vi "MatrixSwitchSingle.vi"(7 "Switch action":u16(ring) items=["Open", "Close"], 8 "error in (no error)":errorcluster, 9 "Matrix Y":i32=1 min=1 max=12 step=1, 10 "Matrix X":i32=1 min=1 max=12 step=1, 11 "LXIPXISwitching in":refnum<class "LXIPXISwitching.lvclass">) -> (0 "error out":errorcluster, 2 "command string":string, 3 "LXIPXISwitching out":refnum<class "LXIPXISwitching.lvclass">)   [LabVIEW 2019, in "LXIPXISwitching.lvclass"]
uses:
  LXIPXISwitching.lvclass
  InstrumentSetup.vi
  InstrControl.lvclass
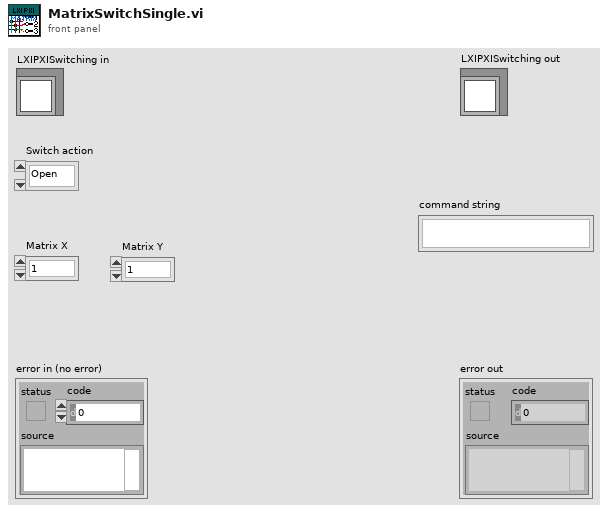
[diagram p1: front panel]
types:
  T1 = cluster{"MUX":string, "Matrix":string, "Breadboard":string, "LXIPXI Switching":refnum<class "LXIPXISwitching.lvclass">, "MUX PN":string, "Matrix  PN":string, "Breadboard PN":string, "MUX ID":string, "Matrix ID":string, "Breadboard ID":string, "LCR?":bool, "SMU?":bool}
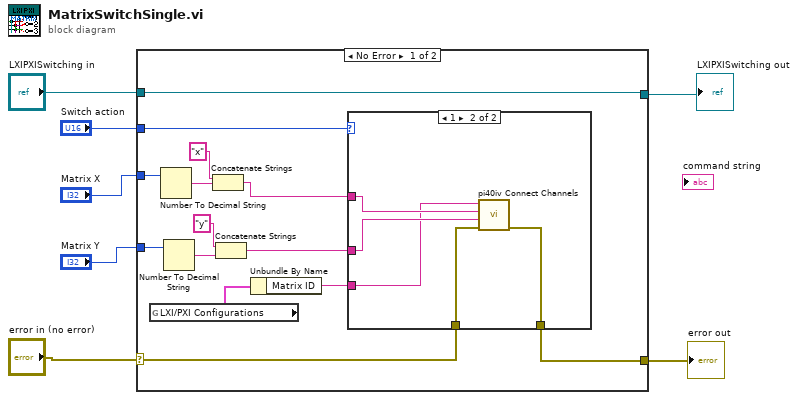
[diagram p0: block diagram]
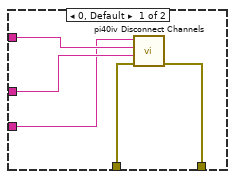
[diagram p2: hidden frame]
diagram:
  n1 = case shown="No Error" "error in (no error)" {
    selector: "error in (no error)" -> [w11 w33]
    tunnel: [w10 w33] -> w6
    tunnel: [w21 w32] -> w4
    tunnel: "LXIPXISwitching in" -> [w21 w32]
    tunnel: "Switch action" -> [w20 _]
    tunnel: "Matrix X" -> [w19 _]
    tunnel: "Matrix Y" -> [w18 _]
    frame No Error {
      n2 = global read "InstrumentSetup.vi" "LXI/PXI Configurations"() -> (w9:T1)
      n3 = Number To Decimal String(number=w19) -> (decimal integer string=w15:string)  [unwired: 1 in]
      n4 = Number To Decimal String(number=w18) -> (decimal integer string=w14:string)  [unwired: 1 in]
      n5 = Concatenate Strings("x" ("string"), w15) -> (w12:string)
      n6 = Concatenate Strings("y" ("string"), w14) -> (w13:string)
      n7 = Unbundle By Name(w9) -> ("Matrix ID"=w8:string)
      n8 = case shown="1" w20 {
        tunnel: w13 -> [w26 w30]
        tunnel: w12 -> [w25 w31]
        tunnel: w11 -> [w24 w29]
        tunnel: [w23 w28] -> w10
        tunnel: w8 -> [w22 w27]
        frame 0, Default {
          n9 = call <instrlib>:"pi40iv Disconnect Channels.vi"("error in (no error)"=w24, "channel 2"=w26, "channel 1"=w25, "instrument handle"=w22) -> ("error out"=w23:errorcluster)  [unwired: 6 in, 1 out]
        }
        frame 1 {
          n10 = call <instrlib>:"pi40iv Connect Channels.vi"("error in (no error)"=w29, "channel 2"=w30, "channel 1"=w31, "instrument handle"=w27) -> ("error out"=w28:errorcluster)  [unwired: 6 in, 1 out]
        }
      }
    }
    frame Error {
    }
  }
  "error out" <- w6
  "LXIPXISwitching out" <- w4
